vi "yaqd_list.vi"(10 "Python path":path=path "C:/ProgramData/Anaconda3/envs/lv4/pythonw.exe") -> (0 "error out":errorcluster, 4 "yaqd list cluster":T1)   [LabVIEW 2022 SP3]
doc: "Lists the host, port, kind, and name of daemons available. Requires path to python associated with an installation of yaqd."
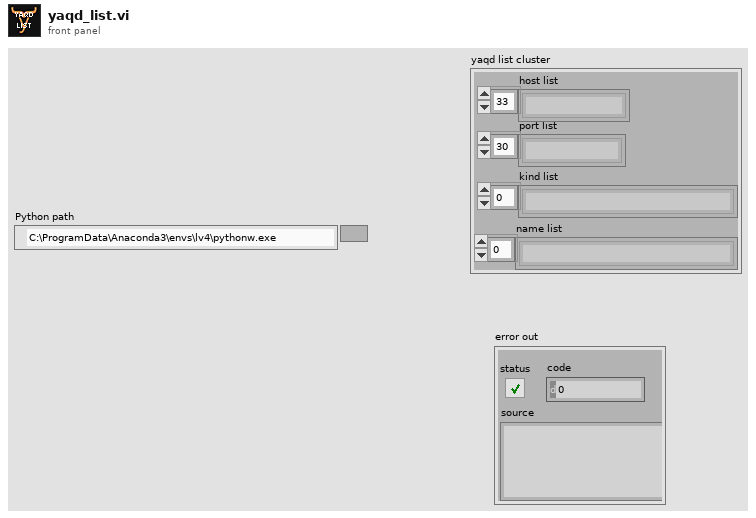
[diagram p1: front panel]
types:
  T1 = cluster{"host list":string[], "port list":string[], "kind list":string[], "name list":string[]}
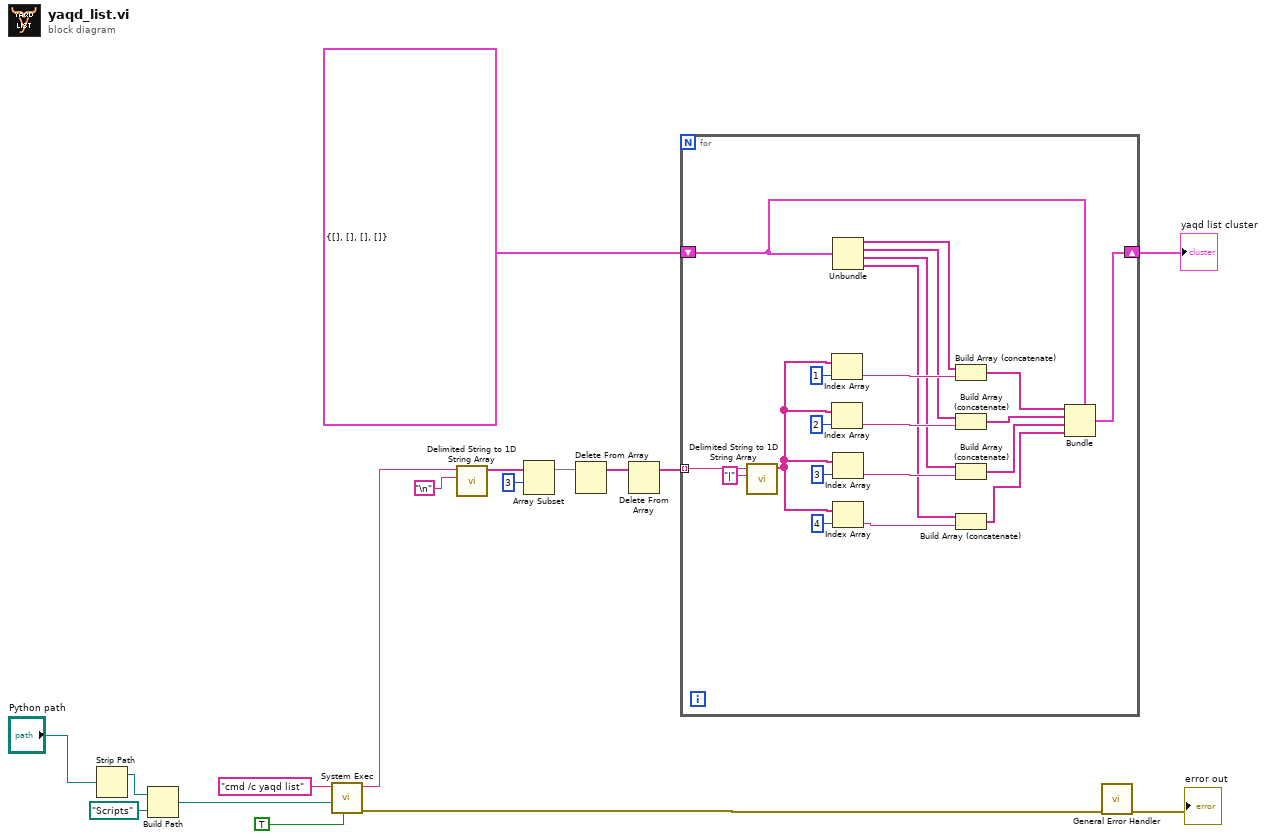
[diagram p0: block diagram]
diagram:
  n1 = Strip Path(path="Python path") -> (stripped path=w14:path)  [unwired: 1 out]
  n2 = Build Path(base path=w14, name or relative path=path "Scripts") -> (appended path=w11:path)
  n3 = call <vilib>:"System Exec.vi"("run minimized? (F)"=TRUE, "working directory"=w11, "command line"="cmd /c yaqd list") -> ("error out"=w16:errorcluster, "standard output"=w9:string)  [unwired: 5 in, 2 out]
  n4 = call <vilib>:"Delimited String to 1D String Array.vi"("delimiter"="\n", "delimited string"=w9) -> ("string array"=w4:string[])  [unwired: 9 in]
  n5 = Array Subset(array=w4, index=3) -> (w5:string[])  [unwired: 1 in]
  n6 = Delete From Array(array=w5) -> (array with subset deleted=w2:string[])  [unwired: 2 in, 1 out]
  n7 = Delete From Array(array=w2) -> (array with subset deleted=w1:string[])  [unwired: 2 in, 1 out]
  n8 = for {
    tunnel: w1 -> [w38] mode=indexing
    shift-right: [w18] -> w6
    shift-left: cluster{string[], string[], string[], string[]} {[], [], [], []} -> [w19]
    n9 = call <vilib>:"Delimited String to 1D String Array.vi"("delimiter"="|", "delimited string"=w38) -> ("string array"=w32:string[])  [unwired: 9 in]
    n10 = Index Array(array=w32, index=1) -> (element=w31:string)
    n11 = Index Array(array=w32, index=2) -> (element=w30:string)
    n12 = Unbundle(w19) -> (w27:string[], w26:string[], w25:string[], w24:string[])
    n13 = Index Array(array=w32, index=3) -> (element=w29:string)
    n14 = Index Array(array=w32, index=4) -> (element=w28:string)
    n15 = Build Array (concatenate)(w27, w31) -> (w23:string[])
    n16 = Build Array (concatenate)(w26, w30) -> (w22:string[])
    n17 = Build Array (concatenate)(w25, w29) -> (w21:string[])
    n18 = Build Array (concatenate)(w24, w28) -> (w20:string[])
    n19 = Bundle(cluster=w19, w23, w22, w21, w20) -> (w18:cluster{string[], string[], string[], string[]})
  }
  "yaqd list cluster" <- w6
  n20 = call <vilib>:"General Error Handler.vi"("error in (no error)"=w16) -> ("error out"=→"error out":errorcluster)  [unwired: 10 in, 4 out]
